vi "Adv_GetControlCurrentCapabilities.vi"(6 "LightField Setting":string, 8 "error in (no error)":errorcluster, 9 "Control Type":refnum<vi>, 10 "Control":refnum<vi>, 11 "LightField Automation in":refnum<class "LightField Automation.lvclass">) -> (0 "error out":errorcluster, 3 "LightField Automation out":refnum<class "LightField Automation.lvclass">)   [LabVIEW 2018, in "LightField Automation.lvclass"]
uses:
  LightField Automation.lvclass
  LightField Automation.lvclass/LightField Automation.ctl
  C:/Users/xw9/Desktop/Turbulence program/SourceDistribution/PrincetonInstruments.LightFieldViewV3.dll
  PrincetonInstruments.LightFieldViewV3.dll
  DialogType.ctl
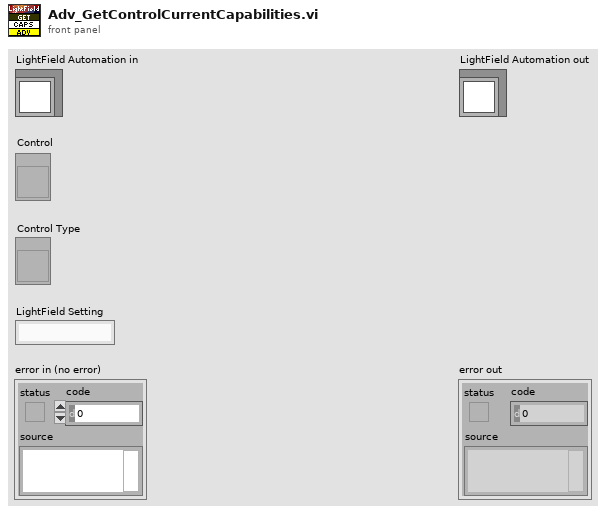
[diagram p1: front panel]
types:
  T1 = typedef "DialogType.ctl" = u16
  T2 = typedef "LVStringsAndValuesArrayTypeDef.ctl" = cluster{"String":string, "Value":ext}[]
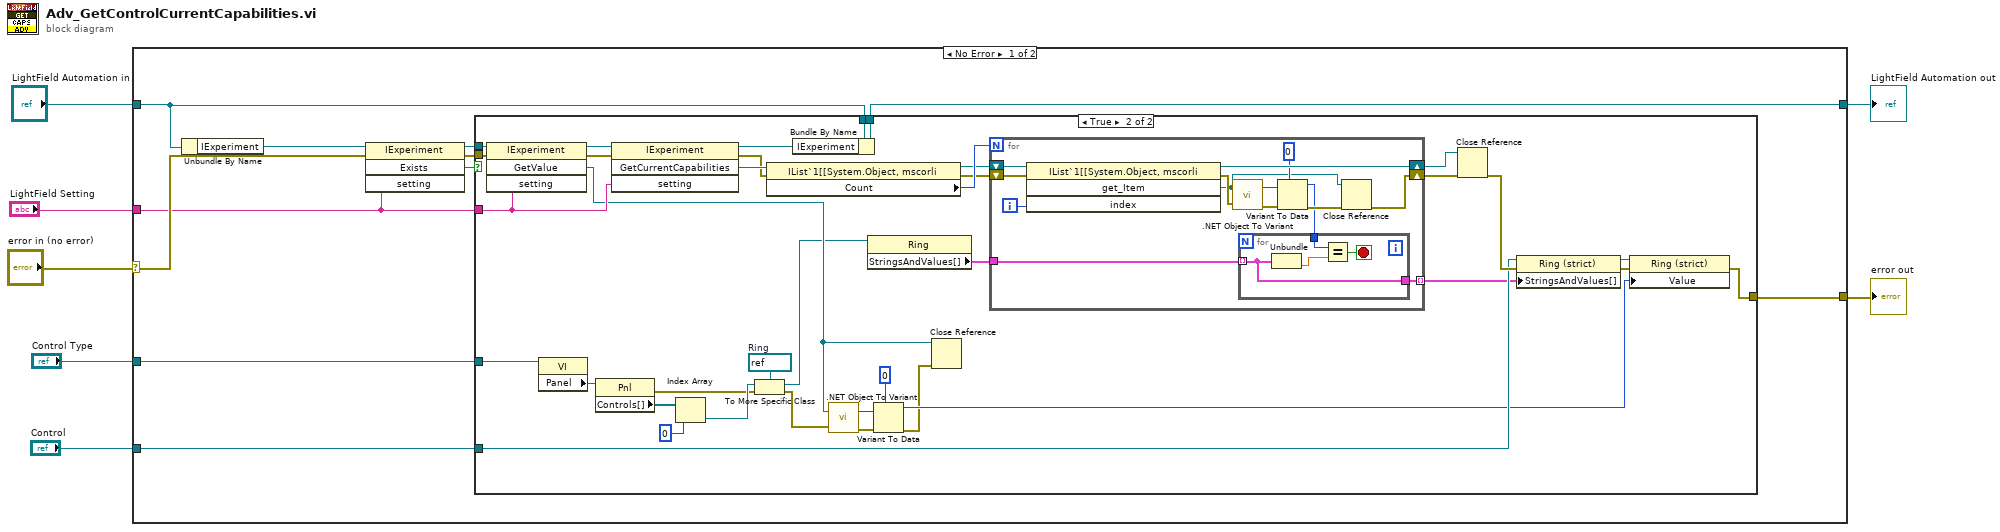
[diagram p0: block diagram]
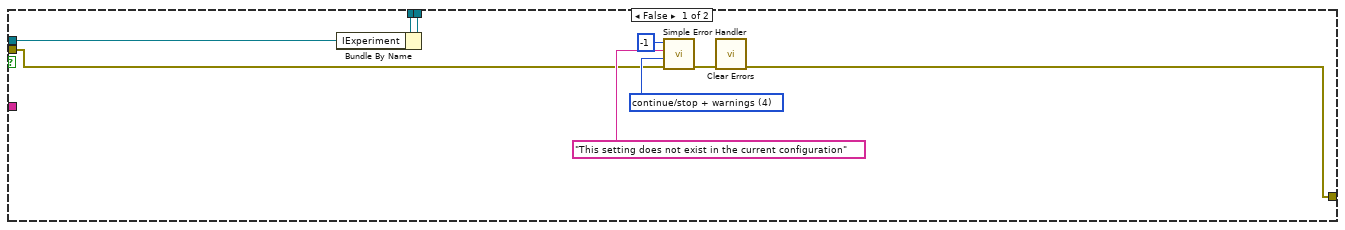
[diagram p2: hidden frame]
diagram:
  n1 = case shown="No Error" "error in (no error)" {
    selector: "error in (no error)" -> [w10 w84]
    tunnel: [w15 w84] -> w6
    tunnel: [w17 w83] -> w4
    tunnel: "LightField Automation in" -> [w18 w83]
    tunnel: "Control" -> [w16 _]
    tunnel: "LightField Setting" -> [w9 _]
    tunnel: "Control Type" -> [w8 _]
    frame No Error {
      n2 = Unbundle By Name(w18) -> ("IExperiment"=w11:refnum<k24>)
      n3 = invoke class="IExperiment" method="Exists"(reference=w11, error in=w10, "setting"=w9) -> (reference out=w13:refnum<k24>, error out=w12:errorcluster, "Exists"=w14:bool)  [unwired: 1 in, 1 out]
      n4 = case shown="True" w14 {
        tunnel: w18 -> [w26 w64]
        tunnel: [w25 w63] -> w17
        tunnel: w16 -> [_ w56]
        tunnel: w13 -> [w27 w52]
        tunnel: w12 -> [w20 w49]
        tunnel: w9 -> [_ w45]
        tunnel: [w19 w38] -> w15
        tunnel: w8 -> [_ w30]
        frame False {
          w21 = T1 4 items=["no dialog", "OK message", "continue or stop message", "OK message + warnings", "continue/stop + warnings"] ("type of dialog (OK msg:1)")
          n5 = Bundle By Name(cluster=w26, "IExperiment"=w27) -> (w25:refnum<class "LightField Automation.lvclass">)
          n6 = call "Simple Error Handler.vi"("error code (no error:0)"=-1, "error source (\" \")"="This setting does not exist in the current configuration" ("source"), "type of dialog (OK msg:1)"=w21, "error in (no error)"=w20) -> ("error out"=w22:errorcluster)  [unwired: 1 in, 4 out]
          n7 = call "Clear Errors.vi"("error in (no error)"=w22) -> ("error out"=w19:errorcluster)  [unwired: 5 in, 1 out]
        }
        frame True {
          w32 = refnum<vi> refnum  # Ring
          n8 = invoke class="IExperiment" method="GetValue"(reference=w52, error in=w49, "setting"=w45) -> (reference out=w51:refnum<k24>, error out=w50:errorcluster, "GetValue"=w40:refnum<k24>)  [unwired: 1 in, 1 out]
          n9 = property class="VI"(reference=w30) -> ("Panel"=w36:refnum<vi>)  [unwired: 1 in, 2 out]
          n10 = property class="Pnl"(reference=w36) -> (error out=w29:errorcluster, "Controls[]"=w35:refnum<vi>[])  [unwired: 1 in, 1 out]
          n11 = invoke class="IExperiment" method="GetCurrentCapabilities"(reference=w51, error in=w50, "setting"=w45) -> (reference out=w55:refnum<k24>, error out=w53:errorcluster, "GetCurrentCapabilities"=w54:refnum<k24>)  [unwired: 1 in, 1 out]
          n12 = Index Array(array=w35, index=0) -> (element=w33:refnum<vi>)
          n13 = To More Specific Class(target class=w32, reference=w33, error in=w29) -> (specific class reference=w31:refnum<vi>, error out=w28:errorcluster)
          n14 = property class="IList`1[[System.Object, mscorli"(reference=w54, error in=w53) -> (reference out=w61:refnum<k24>, error out=w60:errorcluster, "Count"=w62:i32)
          n15 = Bundle By Name(cluster=w64, "IExperiment"=w55) -> (w63:refnum<class "LightField Automation.lvclass">)
          n16 = call ".NET Object To Variant.vi"("error in (no error)"=w28, ".NET object"=w40) -> ("error out"=w48:errorcluster, "variant"=w47:variant)
          n17 = property class="Ring"(reference=w31) -> ("StringsAndValues[]"=w37:T2)  [unwired: 1 in, 2 out]
          n18 = Variant To Data(error in=w48, type=0, Variant=w47) -> (data=w42:i32, error out=w41:errorcluster)
          n19 = Close Reference(reference=w40, error in (no error)=w41) -> ()  [unwired: 1 out]
          n20 = for {
            N: w62 -> [_]
            shift-right: [w75] -> w58
            shift-left: w61 -> [w78]
            shift-right: [w69] -> w59
            shift-left: w60 -> [w77]
            tunnel: w37 -> [w67]
            tunnel: [w65] -> w39 mode=indexing
            i -> [w76]
            n21 = invoke class="IList`1[[System.Object, mscorli" method="get_Item"(reference=w78, error in=w77, "index"=w76) -> (reference out=w75:refnum<k24>, error out=w72:errorcluster, "get_Item"=w68:refnum<k24>)  [unwired: 1 in, 1 out]
            n22 = call ".NET Object To Variant.vi"("error in (no error)"=w72, ".NET object"=w68) -> ("error out"=w74:errorcluster, "variant"=w73:variant)
            n23 = Variant To Data(error in=w74, type=0, Variant=w73) -> (data=w66:i32, error out=w70:errorcluster)
            n24 = for {
              tunnel: w67 -> [w79] mode=indexing
              tunnel: w66 -> [w82]
              tunnel: [w79] -> w65
              stop <- w80 stop-if-true
              n25 = Unbundle(w79) -> ("Value"=w81:ext)  [unwired: 1 out]
              n26 = Equal?(x=w82, y=w81) -> (x = y?=w80:bool)
            }
            n27 = Close Reference(reference=w68, error in (no error)=w70) -> (error out=w69:errorcluster)
          }
          n28 = Close Reference(reference=w58, error in (no error)=w59) -> (error out=w57:errorcluster)
          n29 = property class="Ring (strict)"(reference=w56, error in=w57, "StringsAndValues[]"=w39) -> (reference out=w44:refnum<vi>, error out=w43:errorcluster)
          n30 = property class="Ring (strict)"(reference=w44, error in=w43, "Value"=w42) -> (error out=w38:errorcluster)  [unwired: 1 out]
        }
      }
    }
    frame Error {
    }
  }
  "error out" <- w6
  "LightField Automation out" <- w4
